vi "Main.vi"() -> ()   [LabVIEW 2017, in "Filter Pattern Demo.lvclass"]
uses:
  Filter Pattern Demo.lvclass
  Person Class/Person.lvclass
  AndCriteria Class/AndCriteria.lvclass
  C:/Users/fflores/Documents/LabVIEW-Open-Projects/LabIVEW OOP Design Patterns/Filter Pattern/Criteria Class/Criteria.lvclass
  OrCriteria Class/OrCriteria.lvclass
  CriteriaMale Class/CriteriaMale.lvclass
  CriteriaSingle Class/CiteriaSingle.lvclass
  CriteriaFemale Class/CriteriaFemale.lvclass
  ConsoleOut/Print Options.ctl
  Criteria Class/Criteria.lvclass
panel:
  in  "Raw Data":string[][](table)=[["Robert", "Male", "Single"], ["John", "Male", "Married"], ["Laura", "Female", "Married"], ["Diana", "Female", "Single"], ["Mike", "Male", "Single"], ["Bobby", "Male", "Single"]]
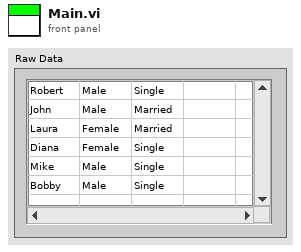
[diagram p1: front panel]
types:
  T1 = typedef "Print Options.ctl" = enum16{"Create", "Get Reference", "Print", "Print Header", "Close"}
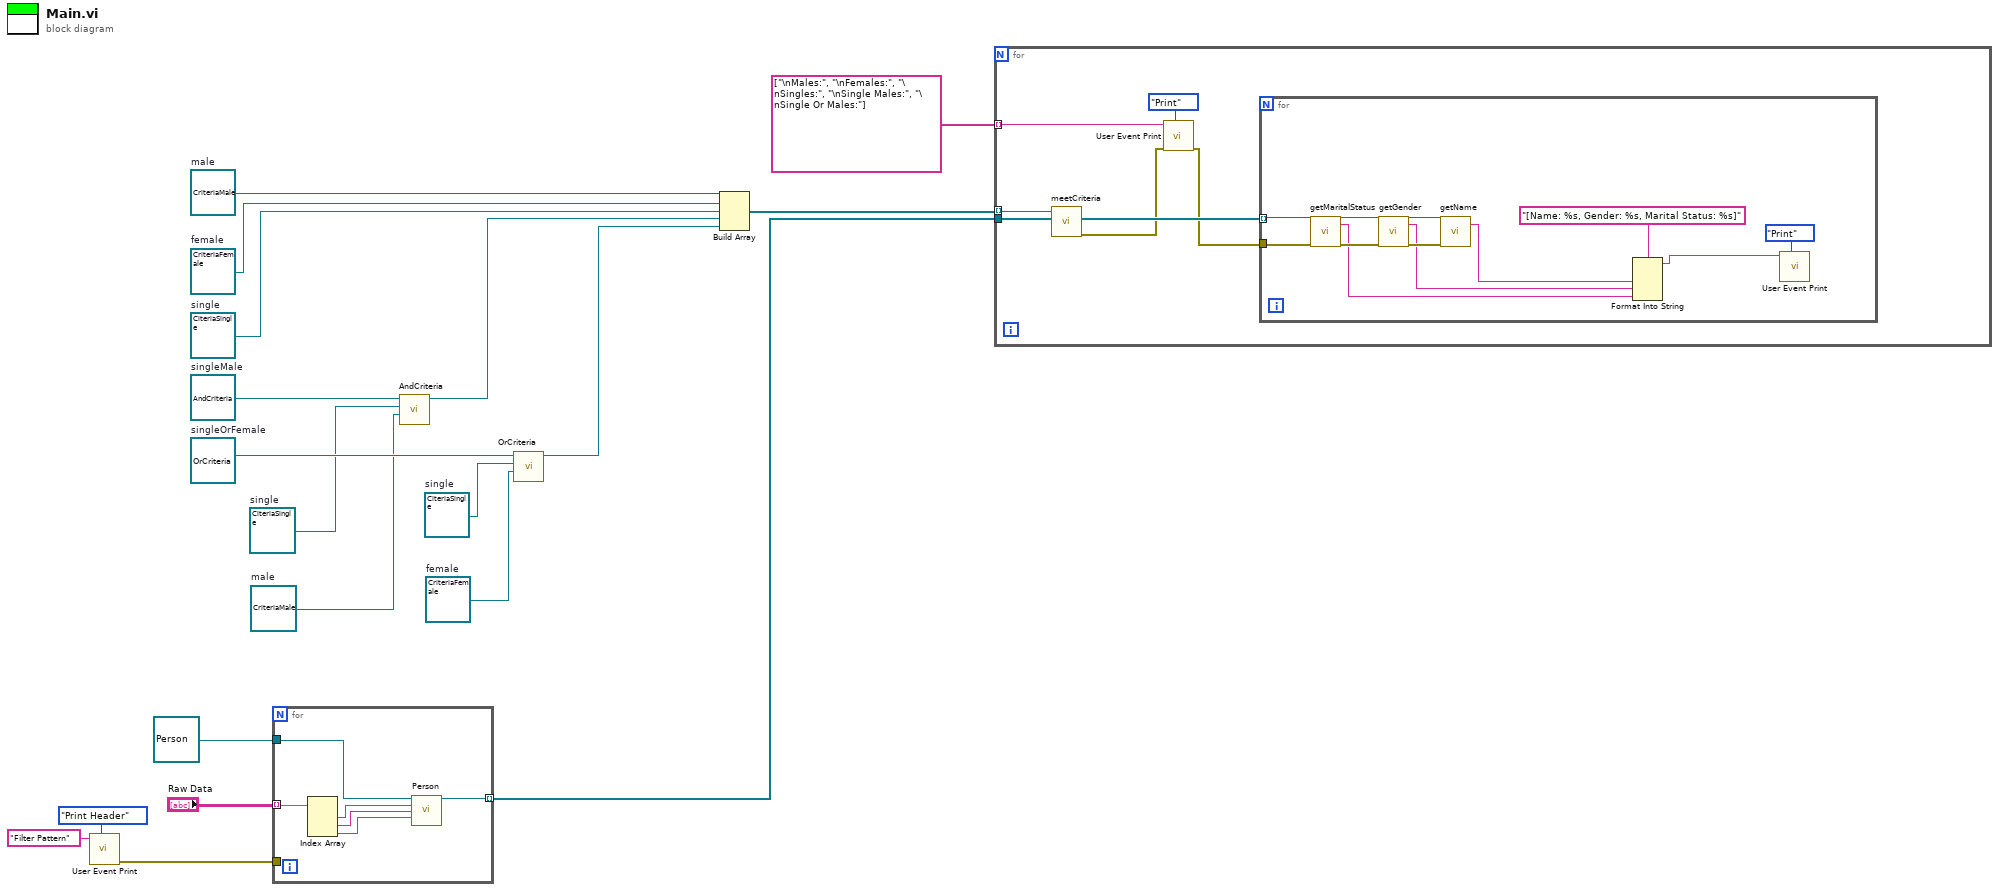
[diagram p0: block diagram]
diagram:
  w13 = refnum<class "CriteriaFemale.lvclass"> refnum  # female
  w14 = refnum<class "CiteriaSingle.lvclass"> refnum  # single
  w15 = refnum<class "CriteriaMale.lvclass"> refnum  # male
  w16 = refnum<class "CiteriaSingle.lvclass"> refnum  # single
  w18 = refnum<class "OrCriteria.lvclass"> refnum  # singleOrFemale
  w17 = refnum<class "AndCriteria.lvclass"> refnum  # singleMale
  w9 = refnum<class "CiteriaSingle.lvclass"> refnum  # single
  w10 = refnum<class "CriteriaFemale.lvclass"> refnum  # female
  w11 = refnum<class "CriteriaMale.lvclass"> refnum  # male
  n1 = call "User Event Print.vi"("Options"=Print_Options."Print Header", "String to Print"="Filter Pattern") -> ("error out"=w2:errorcluster)  [unwired: 8 in, 1 out]
  n2 = for {
    tunnel: "Raw Data" -> [w25] mode=indexing
    tunnel: refnum<class "Person.lvclass"> refnum ("Person.lvclass") -> [w21]
    tunnel: [w20] -> w5 mode=indexing
    tunnel: w2 -> [_]
    n3 = Index Array(array=w25) -> (element #1=w24:string, element #2=w23:string, element #3=w22:string)  [unwired: 3 in]
    n4 = call "Person.vi"("Person in"=w21, "name"=w24, "gender"=w23, "maritalStatus"=w22) -> ("Person out"=w20:refnum<class "Person.lvclass">)  [unwired: 10 in, 1 out]
  }
  n5 = call "AndCriteria.vi"("Other Criteria"=w15, "Criteria"=w16, "AndCriteria in"=w17) -> ("AndCriteria out"=w8:refnum<class "AndCriteria.lvclass">)  [unwired: 7 in, 1 out]
  n6 = call "OrCriteria.vi"("Other Criteria"=w13, "Criteria"=w14, "OrCriteria in"=w18) -> ("OrCriteria out"=w7:refnum<class "OrCriteria.lvclass">)  [unwired: 7 in, 1 out]
  n7 = Build Array(w11, w10, w9, w8, w7) -> (w6:refnum<class "Criteria.lvclass">[])
  n8 = for {
    tunnel: w6 -> [w32] mode=indexing
    tunnel: w5 -> [w31]
    tunnel: string[] ["\nMales:", "\nFemales:", "\nSingles:", "\nSingle Males:", "\nSingle Or Males:"] -> [w27] mode=indexing
    n9 = call-dynamic "meetCriteria.vi"("Persons In"=w31, "Criteria in"=w32) -> ("error out"=w29:errorcluster, "Persons Out"=w30:refnum<class "Person.lvclass">[])  [unwired: 7 in, 1 out]
    n10 = call "User Event Print.vi"("Options"=Print_Options."Print", "error in (no error)"=w29, "String to Print"=w27) -> ("error out"=w28:errorcluster)  [unwired: 7 in, 1 out]
    n11 = for {
      tunnel: w30 -> [w40] mode=indexing
      tunnel: w28 -> [w35]
      n12 = call-dynamic "getMaritalStatus.vi"("error in (no error)"=w35, "Person in"=w40) -> ("error out"=w43:errorcluster, "maritalStatus"=w36:string, "Person out"=w44:refnum<class "Person.lvclass">)  [unwired: 7 in]
      n13 = call-dynamic "getGender.vi"("error in (no error)"=w43, "Person in"=w44) -> ("error out"=w41:errorcluster, "gender"=w37:string, "Person out"=w42:refnum<class "Person.lvclass">)  [unwired: 7 in]
      n14 = call-dynamic "getName.vi"("error in (no error)"=w41, "Person in"=w42) -> ("name"=w38:string)  [unwired: 7 in, 2 out]
      n15 = Format Into String(format string="[Name: %s, Gender: %s, Marital Status: %s]", w38, w37, w36) -> (resulting string=w33:string)  [unwired: 2 in, 1 out]
      n16 = call "User Event Print.vi"("Options"=Print_Options."Print", "String to Print"=w33) -> ()  [unwired: 8 in, 2 out]
    }
  }
